vi "PI Prompt for Prompt Parameters.vi"(8 "error in (no error)":errorcluster, 11 "Results":T1={"Measurement Cycles"=0, "Response"="", "Measurement"={"sxFieldId"="", "sValue"="", "nDataType"=enum."Scalar", "sUnits"="", "sDisplayName"=""}, "Limit"={"Limits On"=TRUE, "Limits"=[]}, "Status Array"=[]}) -> (0 "error out":errorcluster, 3 "Results Out":T1={"Measurement Cycles"=0, "Response"="", "Measurement"={"sxFieldId"="", "sValue"="", "nDataType"=enum."Scalar", "sUnits"="", "sDisplayName"=""}, "Limit"={"Limits On"=TRUE, "Limits"=[]}, "Status Array"=[]})   [LabVIEW 2011]
uses:
  TypeDefs/PI Results.ctl
  TypeDefs/PI Measurement Cluster.ctl
  TypeDefs/PI Limit Parameters.ctl
  TypeDefs/PI Limit Definition.ctl
  TypeDefs/PI Limit Comparison.ctl
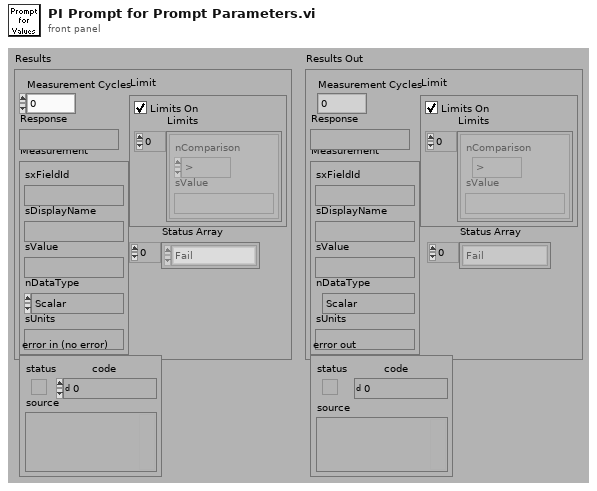
[diagram p1: front panel]
types:
  T1 = typedef "PI Results.ctl" = cluster{"Measurement Cycles":i32, "Response":string, "Measurement":T2, "Limit":T3, "Status Array":enum16{"Fail", "Pass", "Abort", "Error", "Done", "Pass by Sample", "Fail by Sample", "Pass Override", "Fail Override", "Not Tested"}[]}
  T2 = typedef "PI Measurement Cluster.ctl" = cluster{"sxFieldId":string, "sValue":string, "nDataType":enum16{"Scalar", "Enumeration"}, "sUnits":string, "sDisplayName":string}
  T3 = typedef "PI Limit Parameters.ctl" = cluster{"Limits On":bool, "Limits":T4[]}
  T4 = typedef "PI Limit Definition.ctl" = cluster{"nComparison":T5, "sValue":string}
  T5 = typedef "PI Limit Comparison.ctl" = enum16{">", ">=", "<", "<=", "<>", "="}
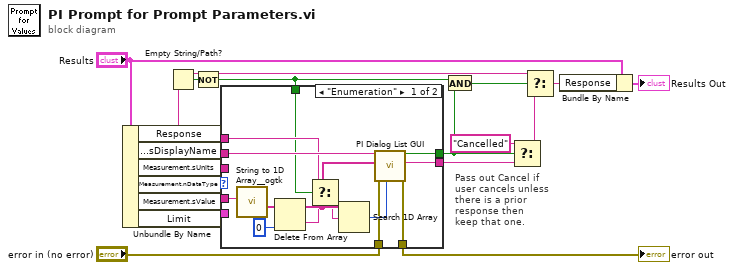
[diagram p0: block diagram]
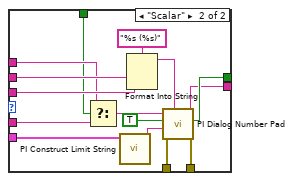
[diagram p2: hidden frame]
diagram:
  # "Pass out Cancel if\nuser cancels unless\nthere is a prior\nresponse then\nkeep that one."
  n1 = Unbundle By Name("Results") -> ("Response"=w2:string, "Measurement.sDisplayName"=w18:string, "Measurement.sUnits"=w4:string, "Measurement.nDataType"=w14:enum16{"Scalar", "Enumeration"}, "Measurement.sValue"=w3:string, "Limit"=w16:T3)
  n2 = Empty String/Path?(string/path=w2) -> (empty?=w13:bool)
  n3 = Not(x=w13) -> (.not. x?=w1:bool)
  n4 = case shown="\"Enumeration\"" w14 {
    tunnel: w18 -> [w27 w45]
    tunnel: w4 -> [_ w44]
    tunnel: [w32 w41] -> w12
    tunnel: [w31 w42] -> w9
    tunnel: w16 -> [_ w40]
    tunnel: "error in (no error)" -> [w28 w38]
    tunnel: [w29 w37] -> w5
    tunnel: w3 -> [w26 w36]
    tunnel: w2 -> [w23 w34]
    tunnel: w1 -> [w20 w33]
    frame "Enumeration" {
      n5 = call "String to 1D Array__ogtk.vi"("string"=w26) -> ("Array of Strings"=w25:string[])  [unwired: 2 in, 8 out]
      n6 = Delete From Array(array=w25, index=0) -> (deleted portion=w22:string, array with subset deleted=w24:string[])  [unwired: 1 in]
      n7 = Select(t=w23, s=w20, f=w22) -> (s? t:f=w21:string)
      n8 = Search 1D Array(1D array=w24, element=w21) -> (index of element=w30:i32)  [unwired: 1 out]
      n9 = call "PI Dialog List GUI.vi"("Select Item"=w30, "error in (no error)"=w28, "List Items"=w24, "Prompt"=w27) -> ("error out"=w29:errorcluster, "Selected List Item"=w32:string, "Cancelled?"=w31:bool)  [unwired: 5 out]
    }
    frame "Scalar" {
      n10 = Select(t=w34, s=w33, f=w36) -> (s? t:f=w35:string)
      n11 = call "PI Construct Limit String.vi"("Limits"=w40) -> ("Limit String"=w39:string)  [unwired: 10 out]
      n12 = Format Into String(format string="%s (%s)", w45, w44) -> (resulting string=w43:string)  [unwired: 2 in, 1 out]
      n13 = call "PI Dialog Number Pad.vi"("Prompt"=w43, "error in (no error)"=w38, "Limit Text"=w39, "Use Decimal? (f)"=TRUE, "Number (\"0.0\")"=w35) -> ("error out"=w37:errorcluster, "Cancelled?"=w42:bool, "Number"=w41:string)  [unwired: 4 out]
    }
  }
  "error out" <- w5
  n14 = And(x=w1, y=w9) -> (x .and. y?=w8:bool)
  n15 = Select(t="Cancelled" ("format string"), s=w9, f=w12) -> (s? t:f=w10:string)
  n16 = Select(t=w2, s=w8, f=w10) -> (s? t:f=w17:string)
  n17 = Bundle By Name(cluster="Results", "Response"=w17) -> (→"Results Out":T1)
